vi "countResult.vi"(10 "pos":i32[][](array[numeric]), 11 "exist":i32[][](array[numeric])) -> (3 "result":i32)   [LabVIEW 2022 SP3, in "subvis.lvlib"]
uses:
  subvis.lvlib
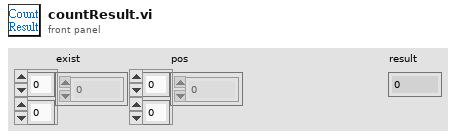
[diagram p1: front panel]
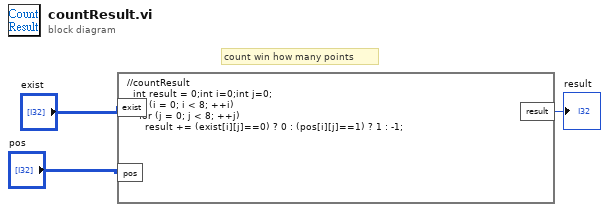
[diagram p0: block diagram]
diagram:
  # "count win how many points"
  n1 = formula code="//countResult\n  int result = 0;int i=0;int j=0;\n  for (i = 0; i < 8; ++i)\n    for (j = 0; j < 8; ++j)\n      result += (exist[i][j]==0) ? 0 : (pos[i][j]==1) ? 1 : -1;"("exist"="exist", "pos"="pos") -> ("result"=→"result":i32)
